vi "Read PORT.vi"(8 "error in (no error)":errorcluster, 11 "Host Adapter in":refnum<class "Host Adapter.lvclass">) -> (0 "error out":errorcluster, 2 "PORT":u16, 3 "Host Adapter out":refnum<class "Host Adapter.lvclass">)   [LabVIEW 2016, in "Host Adapter.lvlib" / "Host Adapter.lvclass"]
uses:
  Host Adapter.lvclass
  Host Adapter.lvclass/Host Adapter.ctl
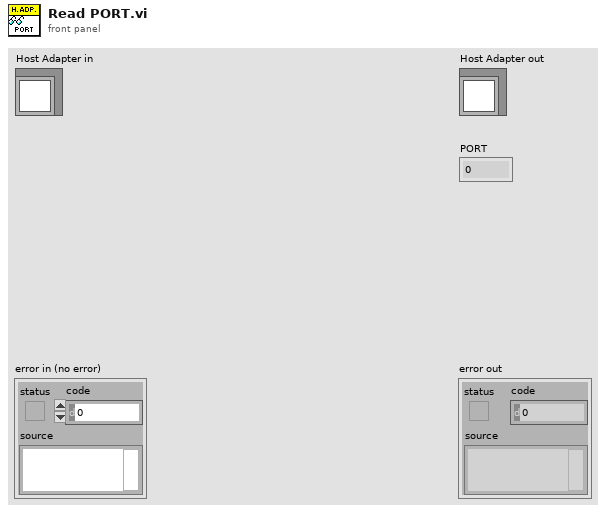
[diagram p1: front panel]
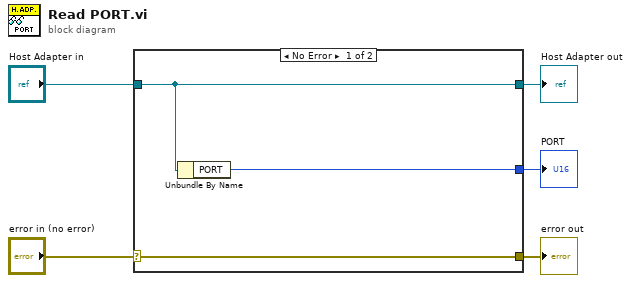
[diagram p0: block diagram]
diagram:
  n1 = case shown="No Error" "error in (no error)" {
    selector: "error in (no error)" -> [w8 w9]
    tunnel: [w8 w9] -> w4
    tunnel: [w7 w10] -> w2
    tunnel: "Host Adapter in" -> [w7 w10]
    tunnel: [w6 _] -> w1
    frame No Error {
      n2 = Unbundle By Name(w7) -> ("PORT"=w6:u16)
    }
    frame Error {
    }
  }
  "error out" <- w4
  "Host Adapter out" <- w2
  "PORT" <- w1
